vi "Splash Screen.vi"() -> ()   [LabVIEW 2013, in "Manager.lvlib"]
doc: "This is the top-level VI of this application. When it runs, it behaves like the splash screen many applications use to keep the user occupied while the application loads into memory. This application is quite small, so there is little overhead, which would make the splash screen just flash for a moment. Because that flash is distracting, there is a three-second delay inserted into this VI so that it stays up for a little bit. \n\nThis VI uses a delay-loaded subVI call to load the rest of the application. This trick ensures that the splash screen can load instantly regardless of how large the rest of the VI hierarchy gets, and the loading of the rest of the VIs becomes one step in the load process."
uses:
  Manager.lvlib
  Load App.vi
  Manager.lvclass
panel:
  out "Application Name":string
  out "Current action:":string
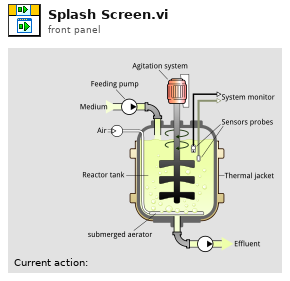
[diagram p1: front panel]
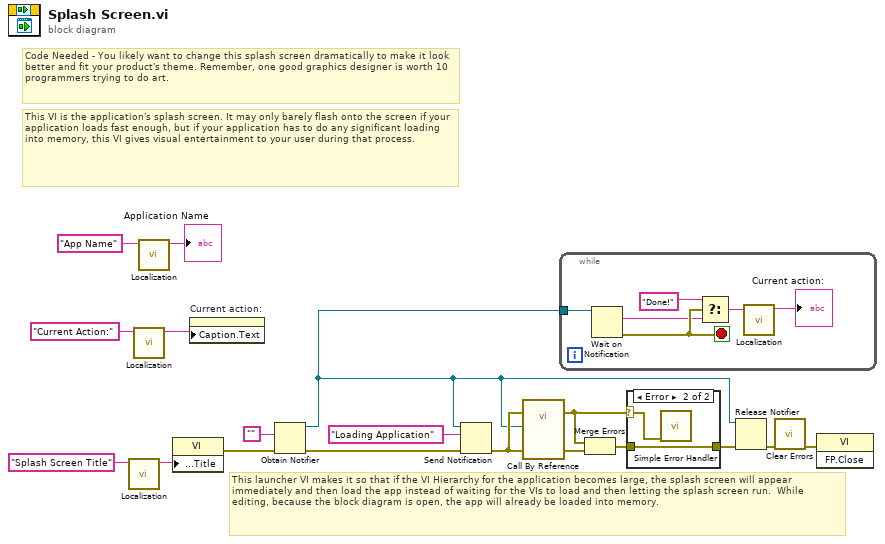
[diagram p0: block diagram]
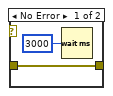
[diagram p2: hidden frame]
diagram:
  # "Code Needed - You likely want to change this splash screen dramatically to make it look better and fit your product's theme. Remember, one good graphics designer is worth 10 programmers trying to do art."
  # "This VI is the application's splash screen. It may only barely flash onto the screen if your application loads fast enough, but if your application has to do any significant loading into memory, this VI gives visual entertainment to your user during that process."
  # "This launcher VI makes it so that if the VI Hierarchy for the application becomes large, the splash screen will appear immediately and then load the app instead of waiting for the VIs to load and then letting the splash screen run.  While editing, because the block diagram is open, the app will already be loaded into memory."
  n1 = call "Localization.vi"("Unlocalized"="Splash Screen Title" ("Window Title")) -> ("Localized"=w18:string)  [unwired: 10 in]
  n2 = call "Localization.vi"("Unlocalized"="Current Action:" ("Window Title")) -> ("Localized"=w4:string)  [unwired: 10 in]
  n3 = call "Localization.vi"("Unlocalized"="App Name") -> ("Localized"=→"Application Name":string)  [unwired: 10 in]
  n4 = property class="VI"("Front Panel.Title"=w18) -> (error out=w16:errorcluster)  [unwired: 2 in, 1 out]
  n5 = property on="Current action:" class="Str"("Caption.Text"=w4) -> ()  [unwired: 2 in, 2 out]
  n6 = Obtain Notifier(notification data type="", error in (no error)=w16) -> (notifier out=w11:refnum<notifier>, error out=w6:errorcluster)  [unwired: 2 in, 1 out]
  n7 = Send Notification(notification="Loading Application", notifier=w11, error in (no error)=w6) -> (error out=w12:errorcluster)  [unwired: 1 out]
  n8 = call-by-ref "?"(error in=w12, 8:"error in (no error)"=w12, "Status Notifier"=w11) -> (error out=w1:errorcluster, 0:"error out"=w15:errorcluster)  [unwired: 10 in, 1 out]
  n9 = while {
    tunnel: w11 -> [w23]
    stop <- w22 stop-if-true
    n10 = Wait on Notification(notifier=w23) -> (notification=w20:string, error out=w22:errorcluster)  [unwired: 3 in, 2 out]
    n11 = Select(t="Done!" ("notification"), s=w22, f=w20) -> (s? t:f=w19:string)
    n12 = call "Localization.vi"("Unlocalized"=w19) -> ("Localized"=→"Current action:":string)  [unwired: 10 in]
  }
  n13 = Merge Errors(w1, w15) -> (w2:errorcluster)
  n14 = case shown="Error" w1 {
    tunnel: [w26 w27] -> w3
    tunnel: w2 -> [w26 w27]
    selector: w1 -> [_ w28]
    frame No Error {
      n15 = Wait (ms)(milliseconds to wait=u32 3000) -> ()  [unwired: 1 out]
    }
    frame Error {
      n16 = call <vilib>:"Simple Error Handler.vi"("error in (no error)"=w28) -> ()  [unwired: 4 in, 5 out]
    }
  }
  n17 = Release Notifier(notifier=w11, error in (no error)=w3) -> (error out=w14:errorcluster)  [unwired: 1 in, 2 out]
  n18 = call <vilib>:"Clear Errors.vi"("error in (no error)"=w14) -> ("error out"=w7:errorcluster)  [unwired: 6 in]
  n19 = invoke class="VI" method="FP.Close"(error in=w7) -> ()  [unwired: 2 in, 3 out]
